vi "SAOMM-XML2LUT.vi"(7 "Path":path) -> (6 "NominalPositions":dbl[](array[numeric]) format="%.6f", 10 "CompleteLUT":dbl[][](array[numeric]))   [LabVIEW 2019]
uses:
  <resource>/objmgr/DOMUserDefRef.rc
  <vilib>/xml/NI_XML.lvlib
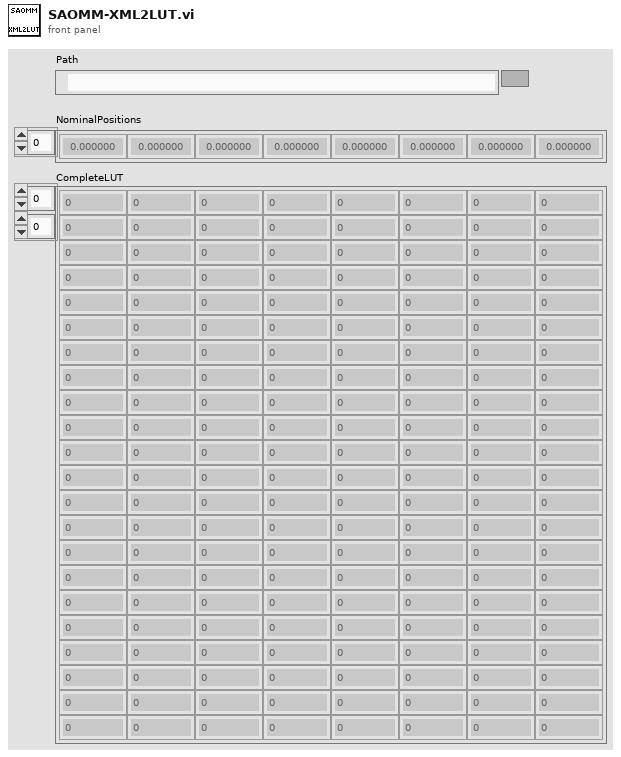
[diagram p1: front panel]
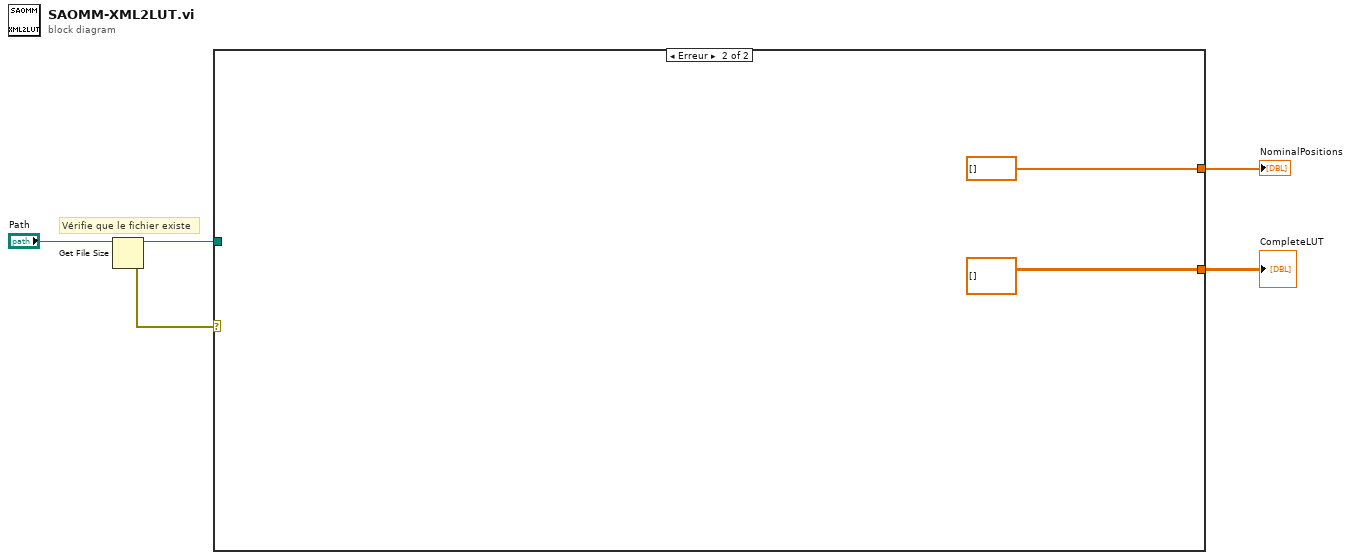
[diagram p0: block diagram]
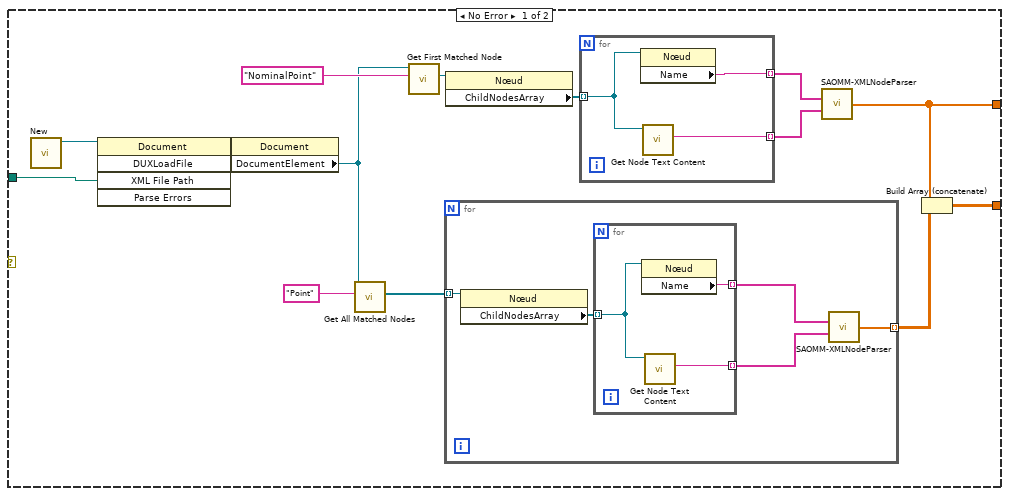
[diagram p2: hidden frame]
diagram:
  # "Vérifie que le fichier existe"
  n1 = Get File Size(file="Path") -> (0:w3:errorcluster)  [unwired: 1 in, 2 out]
  n2 = case shown="Erreur" w3 {
    tunnel: "Path" -> [w12 _]
    tunnel: [w7 dbl[] [] ("PointData")] -> w1
    tunnel: [w6 dbl[][] []] -> w2
    frame No Error {
      n3 = call <vilib>:"New.vi"() -> ("DOM document out"=w18:refnum<k20>)  [unwired: 8 in, 1 out]
      n4 = invoke class="Document" method="DUXLoadFile"(reference=w18, "XML File Path"=w12) -> (reference out=w5:refnum<k20>)  [unwired: 3 in, 4 out]
      n5 = property class="Document"(reference=w5) -> ("DocumentElement"=w11:refnum<k20>)  [unwired: 1 in, 2 out]
      n6 = call <vilib>:"Get All Matched Nodes.vi"("XPath expression"="Point" ("Tag Name"), "node in"=w11) -> ("node result array"=w9:refnum<k20>[])  [unwired: 7 in, 2 out]
      n7 = call <vilib>:"Get First Matched Node.vi"("XPath expression"="NominalPoint" ("Tag Name"), "node in"=w11) -> ("node result"=w15:refnum<k20>)  [unwired: 7 in, 2 out]
      n8 = for {
        tunnel: w9 -> [w23] mode=indexing
        tunnel: [w19] -> w8 mode=indexing
        n9 = property class="Nœud"(reference=w23) -> ("ChildNodesArray"=w22:refnum<k20>[])  [unwired: 1 in, 2 out]
        n10 = for {
          tunnel: [w26] -> w21 mode=indexing
          tunnel: [w25] -> w20 mode=indexing
          tunnel: w22 -> [w24] mode=indexing
          n11 = property class="Nœud"(reference=w24) -> ("Name"=w25:string)  [unwired: 1 in, 2 out]
          n12 = call <vilib>:"Get Node Text Content.vi"("node in"=w24) -> ("node text"=w26:string)  [unwired: 8 in, 2 out]
        }
        n13 = call "SAOMM-XMLNodeParser.vi"("NodeName"=w20, "Node Text"=w21) -> ("PointData"=w19:dbl[])  [unwired: 13 in]
      }
      n14 = property class="Nœud"(reference=w15) -> ("ChildNodesArray"=w16:refnum<k20>[])  [unwired: 1 in, 2 out]
      n15 = for {
        tunnel: w16 -> [w27] mode=indexing
        tunnel: [w29] -> w14 mode=indexing
        tunnel: [w28] -> w13 mode=indexing
        n16 = property class="Nœud"(reference=w27) -> ("Name"=w28:string)  [unwired: 1 in, 2 out]
        n17 = call <vilib>:"Get Node Text Content.vi"("node in"=w27) -> ("node text"=w29:string)  [unwired: 8 in, 2 out]
      }
      n18 = call "SAOMM-XMLNodeParser.vi"("NodeName"=w13, "Node Text"=w14) -> ("PointData"=w7:dbl[])  [unwired: 13 in]
      n19 = Build Array (concatenate)(w7, w8) -> (w6:dbl[][])
    }
    frame Error {
    }
  }
  "NominalPositions" <- w1
  "CompleteLUT" <- w2
